vi "GraspMapContact (SubVI).vi"(1 "position Vector":dbl[](array[numeric]), 2 "r matrix":T1) -> (0 "contact grasp map matrix":T1)   [LabVIEW 2021]
uses:
  <vilib>/Analysis/Matrix/Datatypes/RealMatrix.ctl
  <vilib>/Analysis/baseanly.llb/Real A x B.vi
  <vilib>/Analysis/Matrix/NI_Matrix.lvlib
  <vilib>/Analysis/NI_AALBase.lvlib
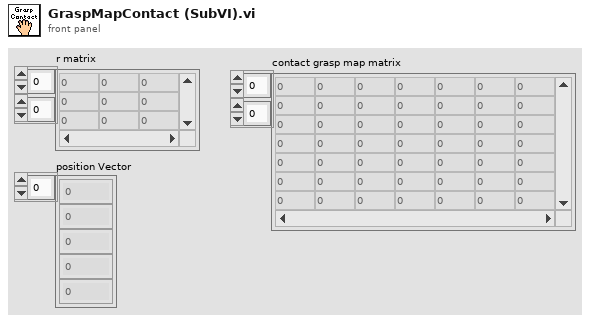
[diagram p1: front panel]
types:
  T1 = typedef "NI_Matrix.lvlib/RealMatrix.ctl" = dbl[][]
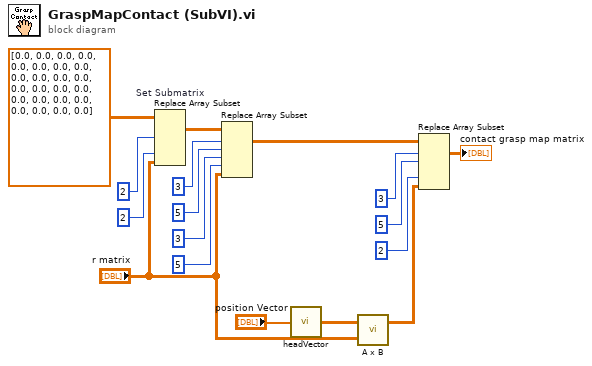
[diagram p0: block diagram]
diagram:
  n1 = Replace Array Subset "Set Submatrix"(array=T1 [[0.0, 0.0, 0.0, 0.0], [0.0, 0.0, 0.0, 0.0], [0.0, 0.0, 0.0, 0.0], [0.0, 0.0, 0.0, 0.0], [0.0, 0.0, 0.0, 0.0], [0.0, 0.0, 0.0, 0.0]] ("matrix"), new element="r matrix", index (dim 1)=2 ("row N"), index (dim 3)=2 ("column N")) -> (w5:T1)  [unwired: 2 in]
  n2 = Replace Array Subset(array=w5, new element="r matrix", index (dim 0)=3 ("row 1"), index (dim 1)=5 ("row N"), index (dim 2)=3 ("column 1"), index (dim 3)=5 ("column N")) -> (w10:T1)
  n3 = call "headVector.vi"("vector"="position Vector") -> ("vector hat"=w14:T1)
  n4 = call-poly <vilib>:"A x B.vi"("B"="r matrix", "A"=w14) -> ("A x B"=w15:T1)  [unwired: 1 out]
  n5 = Replace Array Subset(array=w10, new element=w15, index (dim 0)=3 ("row 1"), index (dim 1)=5 ("row N"), index (dim 3)=2 ("column N")) -> (→"contact grasp map matrix":T1)  [unwired: 1 in]
